vi "test_Read SGL Register Value.vi"(8 "error in (no error)":errorcluster, 11 "TestCase in":refnum<class "FPGA Register IO Tests.lvclass">=refnum) -> (0 "error out":errorcluster, 3 "TestCase out":refnum<class "FPGA Register IO Tests.lvclass">)   [LabVIEW 2026, in "FPGA Register IO Tests.lvclass"]
uses:
  FPGA Register IO Tests.lvclass
  FPGA Register IO Tests.lvclass/FPGA Register IO Tests.ctl
  APIs/FPGA Register IO/FPGA Register IO.lvlib
  <vilib>/rvi/interface/nirviCloseFPGA/nirviCloseFPGA.xnode
  <vilib>/FPGAPlugInAG/Dynamic/niLvFpga_Close_Dynamic.vi
  APIs/FPGA Register IO/Read Methods/Read Data Register/Instances/Read SGL.vi
  Addon/Addon Engine/FPGA Addon Engine.lvlib
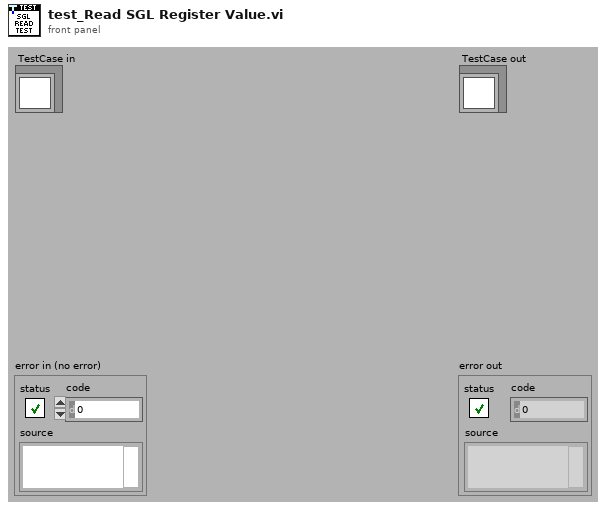
[diagram p1: front panel]
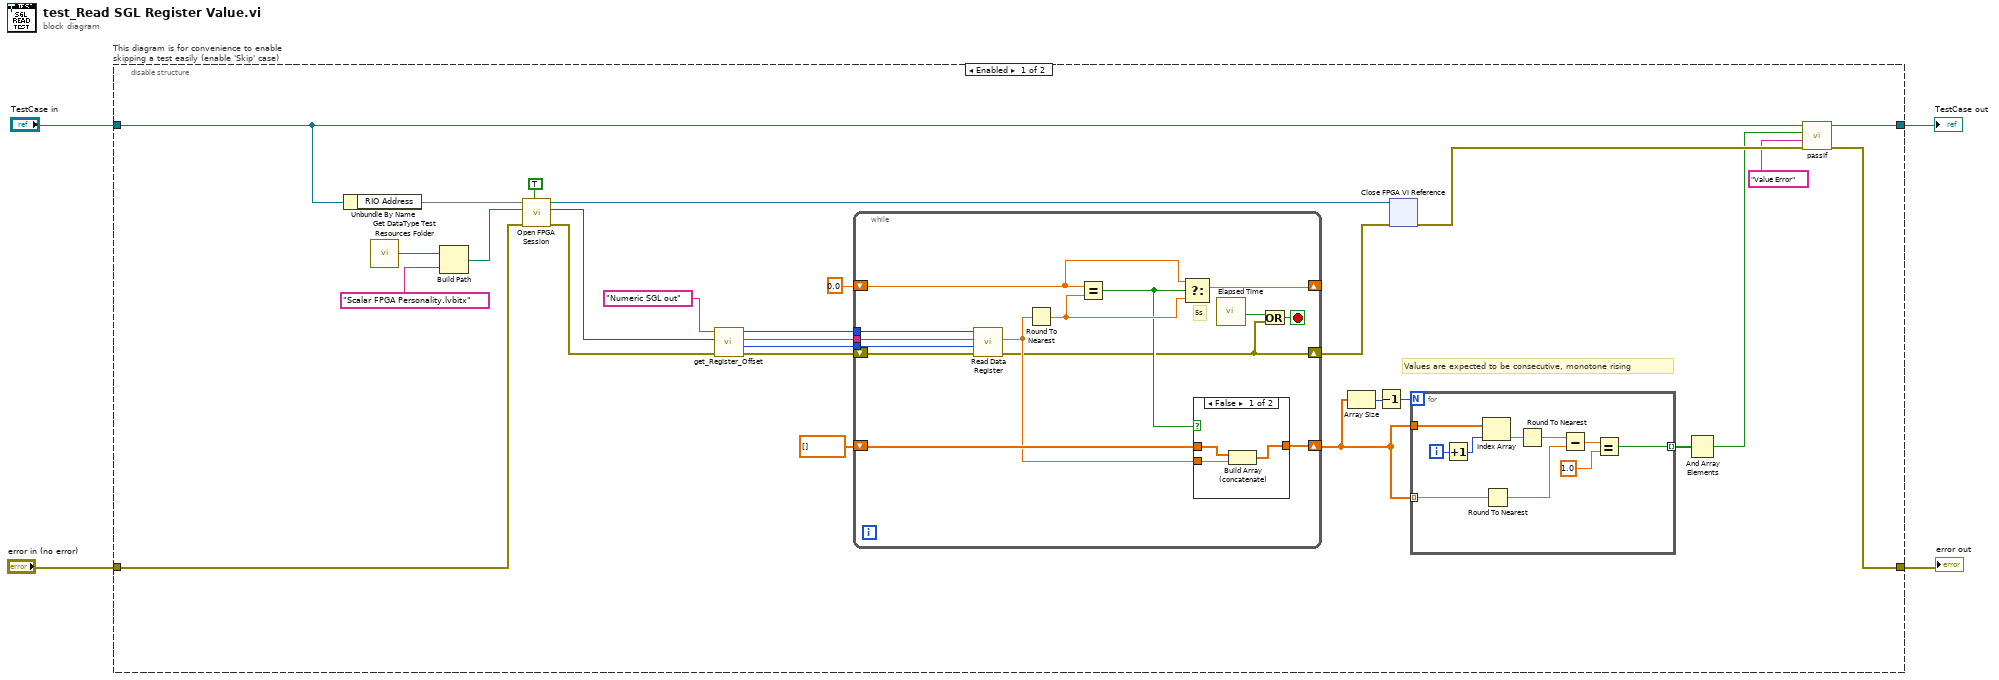
[diagram p0: block diagram]
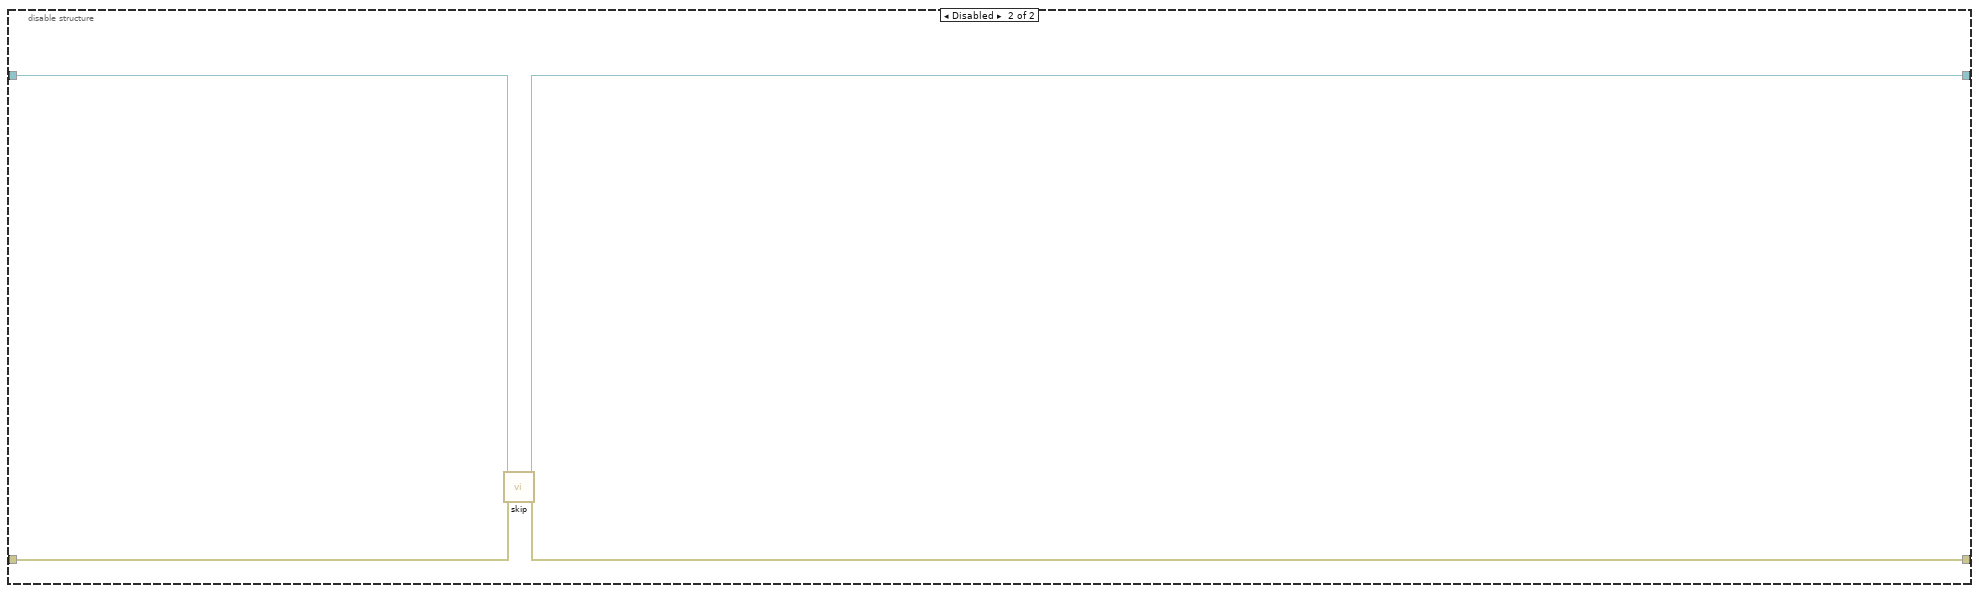
[diagram p3: hidden frame]
diagram:
  n1 = disable-structure "This diagram is for convenience to enable skipping a test easily (enable 'Skip' case)" shown="Enabled" {
    disable-tunnel: "TestCase in" -> [w18 w63]
    disable-tunnel: [w12 w61] -> w1
    disable-tunnel: [w11 w62] -> w3
    disable-tunnel: "error in (no error)" -> [w19 w60]
    frame Enabled {
      # "Values are expected to be consecutive, monotone rising"
      n2 = Unbundle By Name(w18) -> ("RIO Address"=w21)
      n3 = call "Get DataType Test Resources Folder.vi"() -> ("path"=w16:path)
      n4 = Build Path(base path=w16, name or relative path="Scalar FPGA Personality.lvbitx") -> (appended path=w20:path)
      n5 = call "Open FPGA Session.vi"("run when loaded (T)"=TRUE ("Run When Loaded (T)"), "error in"=w19, "bitfile path"=w20, "device address"=w21) -> ("error out"=w26:errorcluster, "session out"=w9:u32, "bitfile reference out"=w25:refnum<k20>)  [unwired: 5 in]
      n6 = call "get_Register_Offset.vi"("error in (no error)"=w26, "session"=w9, "Name"="Numeric SGL out" ("registerName")) -> ("error out"=w10:errorcluster, "RegisterOffset"=w5:u32, "Register Name"=w7:string, "session out"=w8:u32)  [unwired: 5 in]
      n7 = while {
        tunnel: w8 -> [w39]
        shift-right: [w34] -> w24
        shift-left: w10 -> [w38]
        shift-right: [w43] -> _
        shift-left: sgl 0.0 ("DBL Value") -> [w45]
        shift-right: [w41] -> w27
        shift-left: sgl[] [] -> [w40]
        tunnel: w7 -> [w33]
        tunnel: w5 -> [w32]
        stop <- w36 stop-if-true
        # "5s"
        n8 = call-poly "Read Data Register.vi"("error in"=w38, "RegisterOffset"=w32, "register name"=w33, "session in"=w39) -> ("error out"=w34:errorcluster, "value out"=w37:sgl)  [unwired: 5 in, 1 out]
        n9 = Round To Nearest(number=w37) -> (nearest integer value=w44:sgl)
        n10 = Equal?(x=w45, y=w44) -> (x = y?=w42:bool)
        n11 = Select(t=w45, s=w42, f=w44) -> (s? t:f=w43:sgl)
        n12 = case shown="False" w42 {
          tunnel: w37 -> [w48 _]
          tunnel: [w47 w49] -> w41
          tunnel: w40 -> [w46 w49]
          frame False {
            n13 = Build Array (concatenate)(w46, w48) -> (w47:sgl[])
          }
          frame True {
          }
        }
        n14 = call "Elapsed Time"() -> ("Time has Elapsed"=w35:bool)  [unwired: 12 in, 7 out]
        n15 = Or(x=w35, y=w34) -> (x .or. y?=w36:bool)
      }
      n16 = Array Size(array=w27) -> (size(s)=w28:i32)
      n17 = Decrement(x=w28) -> (x-1=w29:i32)
      n18 = xnode "Close FPGA VI Reference"("FPGA VI Reference In"=w25, "error in"=w24) -> ("error out"=w17:errorcluster)
      n19 = for {
        N: w29 -> [_]
        tunnel: w27 -> [w54] mode=indexing
        tunnel: w27 -> [w59]
        tunnel: [w50] -> w30 mode=indexing
        i -> [w58]
        n20 = Increment(x=w58) -> (x+1=w57:i32)
        n21 = Index Array(array=w59, index=w57) -> (element=w56:sgl)
        n22 = Round To Nearest(number=w54) -> (nearest integer value=w53:sgl)
        n23 = Round To Nearest(number=w56) -> (nearest integer value=w55:sgl)
        n24 = Subtract(x=w55, y=w53) -> (x-y=w52:sgl)
        n25 = Equal?(x=w52, y=sgl 1.0) -> (x = y?=w50:bool)
      }
      n26 = And Array Elements(Boolean array=w30) -> (logical AND=w15:bool)
      n27 = call-dynamic "passIf.vi"("error in (no error)"=w17, "message (\"\")"="Value Error" ("message (\"\")"), "pass"=w15, "TestCase in"=w18) -> ("error out"=w11:errorcluster, "TestCase out"=w12:refnum<class "FPGA Register IO Tests.lvclass">)  [unwired: 6 in]
    }
    frame Disabled {
      # "skip test result while test is under development"
      n28 = call <vilib>:"skip.vi"("error in (no error)"=w60, "TestCase in"=w63) -> ("error out"=w62:errorcluster, "TestCase out"=w61:refnum<class "FPGA Register IO Tests.lvclass">)  [unwired: 8 in]
    }
  }
  "error out" <- w3
  "TestCase out" <- w1
